vi "SWLDA_통합버전용.vi"(5 "premove":dbl=0.5, 7 "penter":dbl=0.4, 9 "ERP_Nontarget":dbl[][](array[numeric]) format="%0.3f", 11 "ERP_Target":dbl[][](array[numeric]) format="%0.3f") -> (2 "in":dbl[](array[numeric]), 3 "LDA_matrix":T1, 6 "WEIGHT":dbl[](array[numeric]))   [LabVIEW 2014]
uses:
  <vilib>/Analysis/Matrix/Datatypes/RealMatrix.ctl
  <vilib>/Analysis/baseanly.llb/Vector x A.vi
  <vilib>/Analysis/Matrix/Numeric/Conversions/Array To Matrix - RA.vi
  <vilib>/Analysis/Matrix/Numeric/Conversions/Array To Matrix - RA2.vi
  <vilib>/Analysis/Matrix/NI_Matrix.lvlib
  <vilib>/Analysis/NI_AALBase.lvlib
panel:
  out "biase":dbl[](array[numeric])
  out "Nontarget_mean":dbl[](array[numeric])
  out "Target_mean":dbl[](array[numeric])
  out "Label":dbl[](array[numeric])
  out "Weight":dbl[](array[numeric])
  # "Target/Non-Target of MATLAB"
  # "var_argin part of MATLAB"
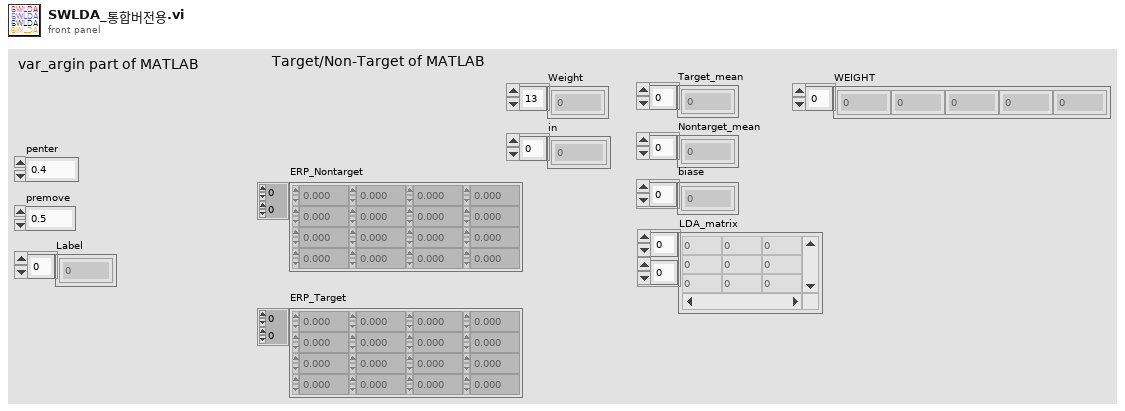
[diagram p1: front panel]
types:
  T1 = typedef "NI_Matrix.lvlib/RealMatrix.ctl" = dbl[][]
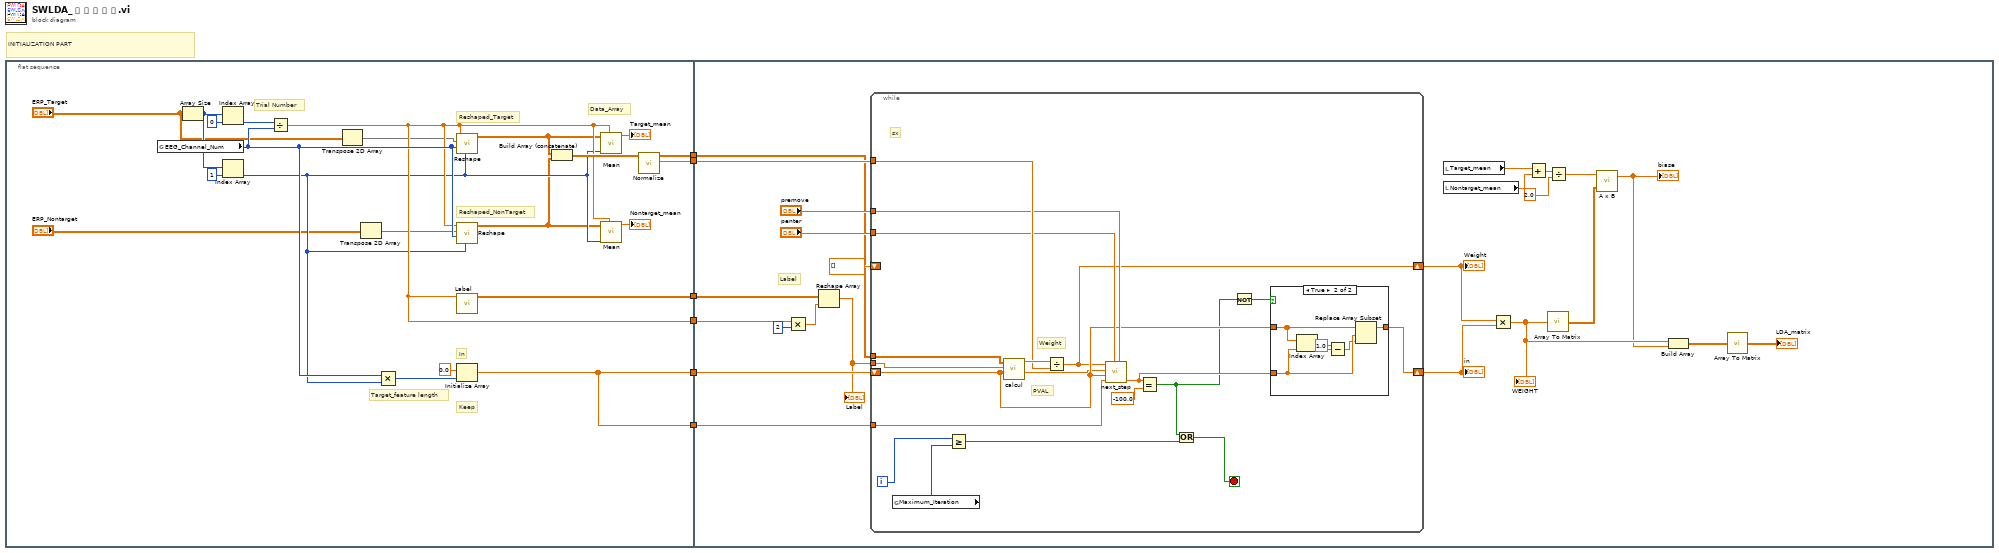
[diagram p0: block diagram]
diagram:
  # "INITIALIZATION PART"
  n1 = flat-sequence {
    tunnel: [w17] -> w6
    tunnel: [w17] -> w5
    tunnel: [w21] -> w4
    tunnel: [w20] -> w3
    tunnel: [w19] -> w2
    tunnel: [w15] -> w1
    tunnel: w6 -> [w51]
    tunnel: w5 -> [w46]
    tunnel: w4 -> [w52]
    tunnel: w3 -> [w42]
    tunnel: w2 -> [w49]
    tunnel: w1 -> [w41]
    frame #0 {
      # "Keep"
      # "In"
      # "Target_feature length"
      # "Data_Array"
      # "Reshaped_NonTarget"
      # "Reshaped_Target"
      # "Trial Number"
      n2 = global read "Control_Panel.vi" "EEG_Channel_Num"() -> (w24:i32)
      n3 = Array Size(array="ERP_Target") -> (size(s)=w26:i32[])
      n4 = Index Array(array=w26, index=0) -> (element=w25:i32)
      n5 = Index Array(array=w26, index=1) -> (element=w14:i32)
      n6 = Divide(x=w25, y=w24) -> (x/y=w15:dbl)
      n7 = Transpose 2D Array(2D array="ERP_Target") -> (transposed array=w12:dbl[][])
      n8 = Transpose 2D Array(2D array="ERP_Nontarget") -> (transposed array=w11:dbl[][])
      n9 = Multiply(x=w24, y=w14) -> (x*y=w23:i32)
      n10 = call "Reshape.vi"("Numeric"=w14, "EEG_Channel_Num"=w24, "all rows"=w12, "Numeric 2"=w15) -> ("Array"=w10:dbl[][])  [unwired: 7 in]
      n11 = call "Reshape.vi"("Numeric"=w14, "EEG_Channel_Num"=w24, "all rows"=w11, "Numeric 2"=w15) -> ("Array"=w7:dbl[][])  [unwired: 7 in]
      n12 = call "Label.vi"("Numeric"=w15) -> ("Array"=w21:dbl[][])  [unwired: 10 in]
      n13 = Initialize Array(0.0 ("element"), w23) -> (w17:dbl[])
      n14 = Build Array (concatenate)(w10, w7) -> (w18:dbl[][])
      n15 = call "Mean.vi"("trial_number"=w15, "feature_number"=w14, "Target/NonTarget"=w10) -> ("mean"=→"Target_mean":dbl[])  [unwired: 8 in]
      n16 = call "Mean.vi"("trial_number"=w15, "feature_number"=w14, "Target/NonTarget"=w7) -> ("mean"=→"Nontarget_mean":dbl[])  [unwired: 8 in]
      n17 = call "Normalize.vi"("Data"=w18) -> ("sx"=w19:dbl[], "Data_out"=w20:dbl[][])  [unwired: 8 in, 1 out]
    }
    frame #1 {
      # "Label"
      n18 = Multiply(x=w41, y=2) -> (x*y=w44:dbl)
      n19 = Reshape Array(w52, w44) -> (w50:dbl[])
      "Label" <- w50
      n20 = while {
        shift-right: [w59] -> w33
        shift-left: w51 -> [w60]
        tunnel: w50 -> [w68]
        tunnel: w42 -> [w67]
        tunnel: w49 -> [w65]
        tunnel: "penter" -> [w64]
        tunnel: "premove" -> [w63]
        tunnel: w46 -> [w62]
        shift-right: [w58] -> w34
        shift-left: dbl[] [] -> [_]
        i -> [w71]
        stop <- w69 stop-if-true
        # "sx"
        # "PVAL"
        # "Weight"
        n21 = global read "Control_Panel.vi" "Maximum_Iteration"() -> (w53:i64)
        n22 = Greater Or Equal?(x=w71, y=w53) -> (x >= y?=w70:bool)
        n23 = call "calcul.vi"("In"=w60, "Label (y)"=w68, "Data (allx)"=w67) -> ("PVAL"=w54:dbl[], "B"=w66:dbl[])  [unwired: 7 in]
        n24 = Divide(x=w66, y=w65) -> (x/y=w58:dbl[])
        n25 = call "next_step.vi"("premove"=w63, "penter"=w64, "keep"=w62, "in"=w60, "PVal"=w54, "B"=w58) -> ("swap"=w57:dbl)  [unwired: 4 in, 1 out]
        n26 = Equal?(x=w57, y=-100.0) -> (x = y?=w55:bool)
        n27 = Or(x=w55, y=w70) -> (x .or. y?=w69:bool)
        n28 = Not(x=w55) -> (.not. x?=w56:bool)
        n29 = case shown="True" w56 {
          tunnel: w60 -> [w72 w77]
          tunnel: w57 -> [_ w76]
          tunnel: [w72 w78] -> w59
          frame False {
          }
          frame True {
            n30 = Index Array(array=w77, index=w76) -> (element=w75:dbl)
            n31 = Subtract(x=1.0, y=w75) -> (x-y=w73:dbl)
            n32 = Replace Array Subset(array=w77, new element=w73, index=w76) -> (w78:dbl[])
          }
        }
      }
      "Weight" <- w34
      "in" <- w33
      n33 = local read "Target_mean"() -> (w40:dbl[])
      n34 = local read "Nontarget_mean"() -> (w39:dbl[])
      n35 = Multiply(x=w34, y=w33) -> (x*y=w32:dbl[])
      "WEIGHT" <- w32
      n36 = Add(x=w40, y=w39) -> (x+y=w38:dbl[])
      n37 = call-poly <vilib>:"Array To Matrix.vi"("Real 1D Array"=w32) -> ("Real Matrix (Column Vector)"=w35:T1)
      n38 = Divide(x=w38, y=2.0) -> (x/y=w36:dbl[])
      n39 = call-poly <vilib>:"A x B.vi"("Matrix A"=w35, "Vector V'"=w36) -> ("V' x A"=w31:dbl[])  [unwired: 1 out]
      "biase" <- w31
      n40 = Build Array(w32, w31) -> (w29:dbl[][])
      n41 = call-poly <vilib>:"Array To Matrix.vi"("Real 2D Array"=w29) -> ("Real Matrix"=→"LDA_matrix":T1)
    }
  }
